vi "Alldelete.vi"(0 "Connection ID Out":T1, 7 "Strings":string, 11 "error in (no error)":errorcluster) -> (4 "Connection ID":T1, 15 "error out":errorcluster)   [LabVIEW 2017]
uses:
  Driver/ConnectionID.ctl
  GL860_Driver.lvlib
panel:
  out "Arrays2":string[][](array[string])
  out "Arrays":string[][](array[string])
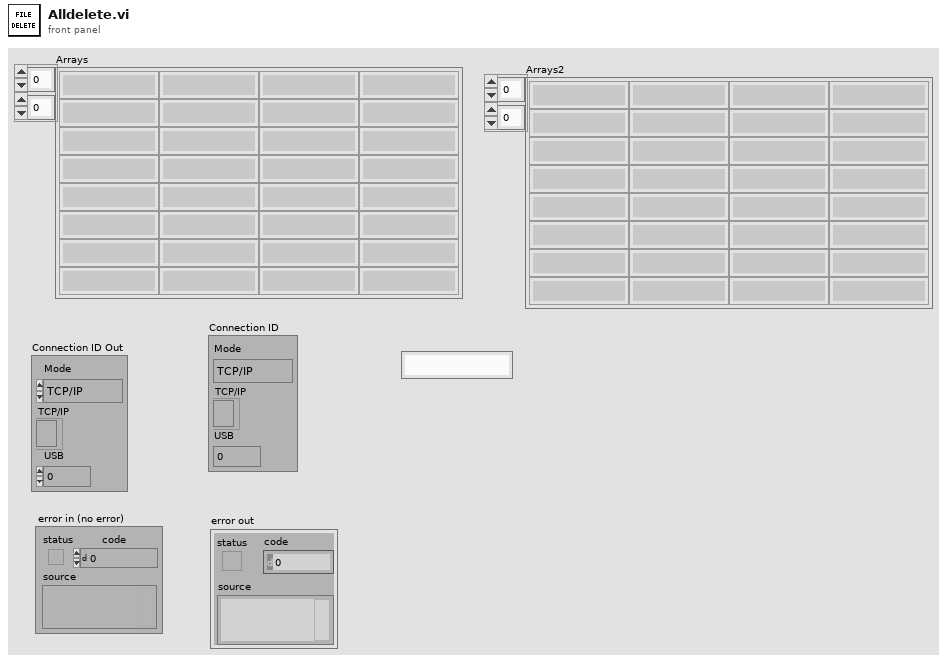
[diagram p1: front panel]
types:
  T1 = typedef "ConnectionID.ctl" = cluster{"Mode":enum16{"TCP/IP", "USB"}, "TCP/IP":refnum<k5>, "USB":i32}
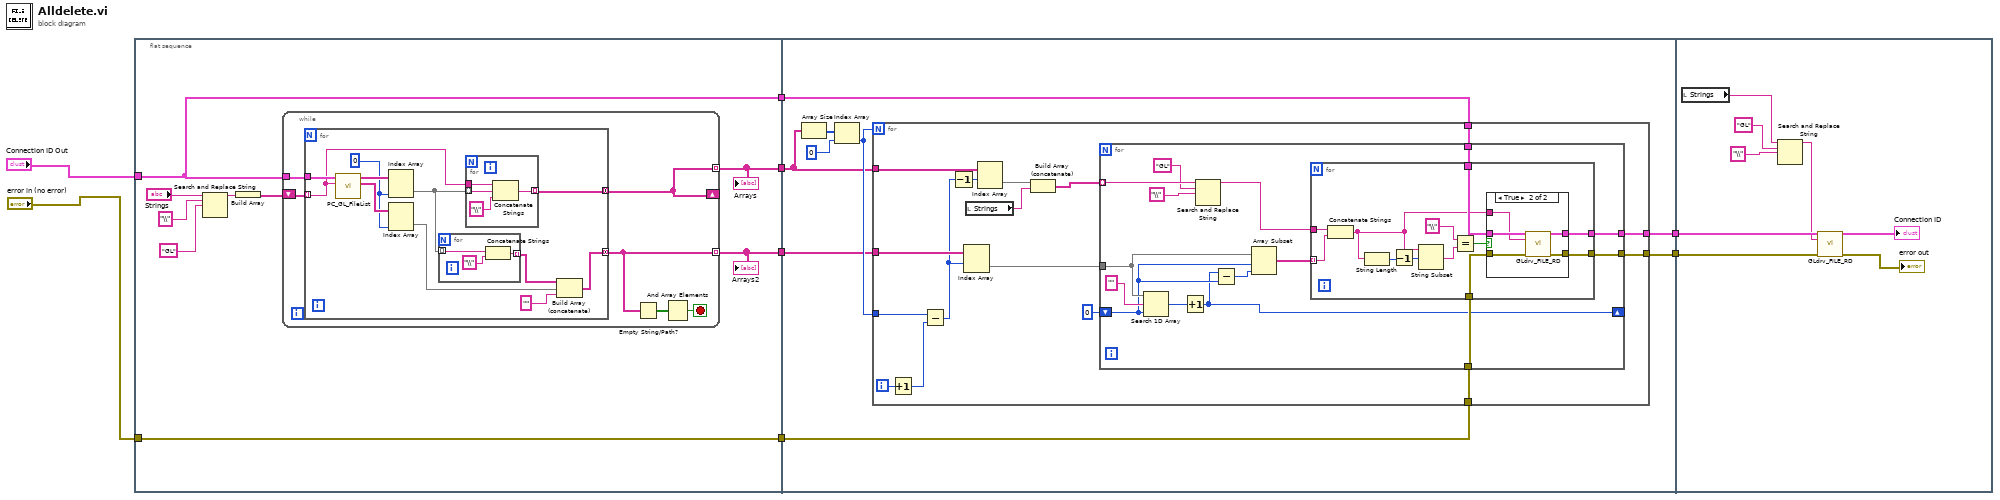
[diagram p0: block diagram]
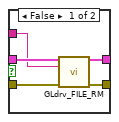
[diagram p2: hidden frame]
diagram:
  n1 = flat-sequence {
    tunnel: "Connection ID Out" -> [w16]
    tunnel: [w16] -> w6
    tunnel: "error in (no error)" -> [w17]
    tunnel: [w17] -> w5
    tunnel: [w14] -> w2
    tunnel: [w13] -> w1
    tunnel: w6 -> [w50]
    tunnel: w5 -> [w47]
    tunnel: [w49] -> w4
    tunnel: [w48] -> w3
    tunnel: w2 -> [w42]
    tunnel: w1 -> [w43]
    tunnel: w4 -> [w111]
    tunnel: w3 -> [w110]
    frame #0 {
      n2 = Search and Replace String(input string="Strings", search string="\\" ("検索文字列"), replace string="GL" ("置換文字列（\"\"）")) -> (result string=w12:string)  [unwired: 5 in, 3 out]
      n3 = Build Array(w12) -> (w15:string[])
      n4 = while {
        tunnel: w16 -> [w22]
        shift-right: [w20] -> _
        shift-left: w15 -> [w23]
        tunnel: [w20] -> w14 mode=indexing
        tunnel: [w19] -> w13 mode=indexing
        stop <- w18 stop-if-true
        n5 = for {
          tunnel: w23 -> [w29] mode=indexing
          tunnel: w22 -> [w34]
          tunnel: [w30] -> w20 mode=concatenating
          tunnel: [w27] -> w19 mode=concatenating
          w31 = 0
          n6 = call "PC_GL_FileList.vi"("Path In"=w29, "Connection ID"=w34) -> ("File"=w32:string[][], "Folder"=w33:string[][])  [unwired: 7 in, 1 out]
          n7 = Index Array(array=w33, index (col)=w31) -> (element=w26:string[])  [unwired: 1 in]
          n8 = Index Array(array=w32, index (col)=w31) -> (element=w28:string[])  [unwired: 1 in]
          n9 = for {
            tunnel: w26 -> [w37] mode=indexing
            tunnel: [w35] -> w25 mode=indexing
            n10 = Concatenate Strings(w37, "\\" ("文字列")) -> (w35:string)
          }
          n11 = for {
            tunnel: w26 -> [w41] mode=indexing
            tunnel: [w39] -> w30 mode=indexing
            tunnel: w29 -> [w38]
            n12 = Concatenate Strings(w38, w41, "\\" ("文字列")) -> (w39:string)
          }
          n13 = Build Array (concatenate)(w25, w28, "" ("要素")) -> (w27:string[])
        }
        n14 = Empty String/Path?(string/path=w19) -> (empty?=w21:bool[])
        n15 = And Array Elements(Boolean array=w21) -> (logical AND=w18:bool)
      }
      "Arrays" <- w14
      "Arrays2" <- w13
    }
    frame #1 {
      n16 = Array Size(array=w42) -> (size(s)=w46:i32[])
      n17 = Index Array(array=w46, index=0 ("指標")) -> (element=w44:i32)
      n18 = for {
        N: w44 -> [_]
        tunnel: w50 -> [w66]
        tunnel: [w65] -> w49
        tunnel: [w64] -> w48
        tunnel: w43 -> [w63]
        tunnel: w42 -> [w62]
        tunnel: w47 -> [w61]
        tunnel: w44 -> [w59]
        i -> [w60]
        n19 = Increment(x=w60) -> (x+1=w57:i32)
        n20 = Subtract(x=w59, y=w57) -> (x-y=w56:i32)
        n21 = Decrement(x=w56) -> (x-1=w58:i32)
        n22 = Index Array(array=w63, index (row)=w56) -> (element=w55:string[])  [unwired: 1 in]
        n23 = local read "Strings"() -> (w51:string)
        n24 = Index Array(array=w62, index (row)=w58) -> (element=w53:string[])  [unwired: 1 in]
        n25 = Build Array (concatenate)(w53, w51) -> (w52:string[])
        n26 = for {
          tunnel: w66 -> [w81]
          tunnel: [w80] -> w65
          tunnel: [w79] -> w64
          tunnel: w61 -> [w78]
          tunnel: w52 -> [w70] mode=indexing
          tunnel: w55 -> [w76]
          shift-right: [w71] -> _
          shift-left: 0 -> [w73]
          n27 = Search 1D Array(1D array=w76, element="" ("要素"), start index (0)=w73) -> (index of element=w74:i32)
          n28 = Increment(x=w74) -> (x+1=w71:i32)
          n29 = Search and Replace String(input string=w70, search string="GL" ("検索文字列"), replace string="\\" ("置換文字列（\"\"）")) -> (result string=w67:string)  [unwired: 5 in, 3 out]
          n30 = Subtract(x=w71, y=w73) -> (x-y=w75:i32)
          n31 = Array Subset(array=w76, index=w73, length=w75) -> (w72:string[])
          n32 = for {
            tunnel: w81 -> [w93]
            tunnel: [w92] -> w80
            tunnel: [w91] -> w79
            tunnel: w78 -> [w90]
            tunnel: w72 -> [w89] mode=indexing
            tunnel: w67 -> [w88]
            n33 = Concatenate Strings(w88, w89) -> (w82:string)
            n34 = String Length(string=w82) -> (length=w87:i32)
            n35 = Decrement(x=w87) -> (x-1=w86:i32)
            n36 = String Subset(string=w82, offset (0)=w86) -> (substring=w84:string)  [unwired: 1 in]
            n37 = Equal?(x="\\", y=w84) -> (x = y?=w85:bool)
            n38 = case shown="TRUE" w85 {
              tunnel: [w98 w100] -> w92
              tunnel: [w97 w101] -> w91
              tunnel: w93 -> [w96 w103]
              tunnel: w90 -> [w95 w102]
              tunnel: w82 -> [w94 w99]
              frame False {
                n39 = call "GLdrv_FILE_RM.vi"("Connection ID"=w96, "File Path"=w94, "error in (no error)"=w95) -> ("Connection ID Out"=w98:T1, "error out"=w97:errorcluster)  [unwired: 11 out]
              }
              frame True {
                n40 = call "GLdrv_FILE_RD.vi"("Connection ID"=w103, "Folder"=w99, "error in (no error)"=w102) -> ("Connection ID Out"=w100:T1, "error out"=w101:errorcluster)  [unwired: 11 out]
              }
            }
          }
        }
      }
    }
    frame #2 {
      n41 = local read "Strings"() -> (w105:string)
      n42 = Search and Replace String(input string=w105, search string="GL" ("検索文字列"), replace string="\\" ("置換文字列（\"\"）")) -> (result string=w104:string)  [unwired: 5 in, 3 out]
      n43 = call "GLdrv_FILE_RD.vi"("Connection ID"=w111, "Folder"=w104, "error in (no error)"=w110) -> ("Connection ID Out"=→"Connection ID":T1, "error out"=→"error out":errorcluster)  [unwired: 11 out]
    }
  }
